vi "动态调用vi.vi"(1 "错误输入（无错误）":errorcluster, 2 "VI路径":path) -> (0 "error out":errorcluster caption="错误输出")   [LabVIEW 2014]
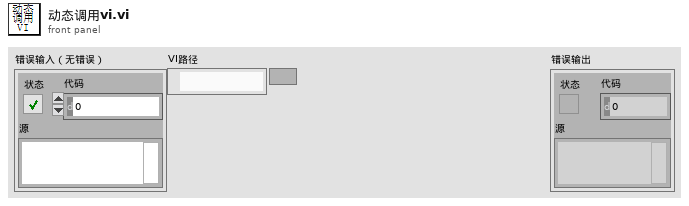
[diagram p1: front panel]
types:
  T1 = enum32{"Invalid", "Standard", "Closed", "Hidden", "Minimized", "Maximized"}
  T2 = enum32{"Bad", "Idle", "Run top level", "Running"}
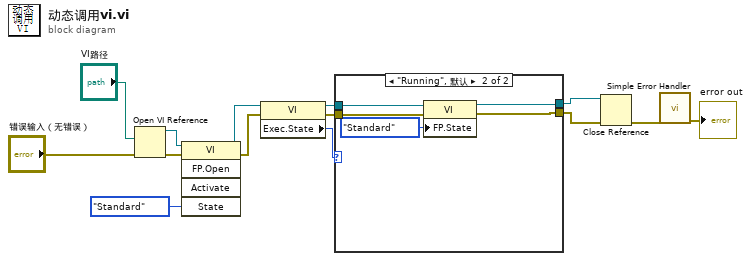
[diagram p0: block diagram]
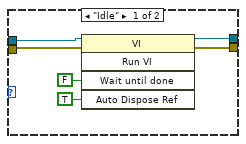
[diagram p2: hidden frame]
diagram:
  n1 = Open VI Reference(vi path="VI路径", error in (no error)="错误输入（无错误）") -> (vi reference=w14:refnum<vi>, error out=w13:errorcluster)  [unwired: 4 in]
  n2 = invoke class="VI" method="FP.Open"(reference=w14, error in=w13, "State"=T1."Standard" ("状态")) -> (reference out=w11:refnum<vi>, error out=w10:errorcluster)  [unwired: 2 in, 3 out]
  n3 = property class="VI"(reference=w11, error in=w10) -> (reference out=w8:refnum<vi>, error out=w7:errorcluster, "Exec.State"=w9:T2)
  n4 = case shown="\"Running\", 默认" w9 {
    tunnel: w8 -> [w18 w25]
    tunnel: w7 -> [w17 w24]
    tunnel: [w16 w22] -> w6
    tunnel: [w15 w21] -> w5
    frame "Idle" {
      n5 = invoke class="VI" method="Run VI"(reference=w18, error in=w17, "Wait until done"=FALSE ("结束前等待"), "Auto Dispose Ref"=TRUE ("自动销毁引用")) -> (reference out=w16:refnum<vi>, error out=w15:errorcluster)  [unwired: 1 in, 3 out]
    }
    frame "Running", Default {
      n6 = property class="VI"(reference=w25, error in=w24, "FP.State"=T1."Standard" ("前面板窗口:状态")) -> (reference out=w22:refnum<vi>, error out=w21:errorcluster)
    }
  }
  n7 = Close Reference(reference=w6, error in (no error)=w5) -> (error out=w4:errorcluster)
  n8 = call <vilib>:"Simple Error Handler.vi"("error in (no error)"=w4) -> ("error out"=→"error out":errorcluster)  [unwired: 4 in, 4 out]
